vi "_PC_RTcheck rt_work_state.vi"(8 "error in (no error)":errorcluster, 11 "Stop":refnum<vi>) -> (0 "error out":errorcluster)   [LabVIEW 2018]
uses:
  RT/PublicSubVI/Ctl/_ctl_RT_Working_State.ctl
  <vilib>/Platform/TimedLoop/XDataNode/timing_clust.ctl
  <vilib>/Platform/TimedLoop/XDataNode/nitl_modes.ctl
  <vilib>/Platform/TimedLoop/XDataNode/wakeup.ctl
  <vilib>/Platform/TimedLoop/XDataNode/XDataNode.xnode
  <resource>/objmgr/ni.var.rc
  <vilib>/Platform/TimedLoop/XDataNode/XDNodeRunTimeDep.lvlib
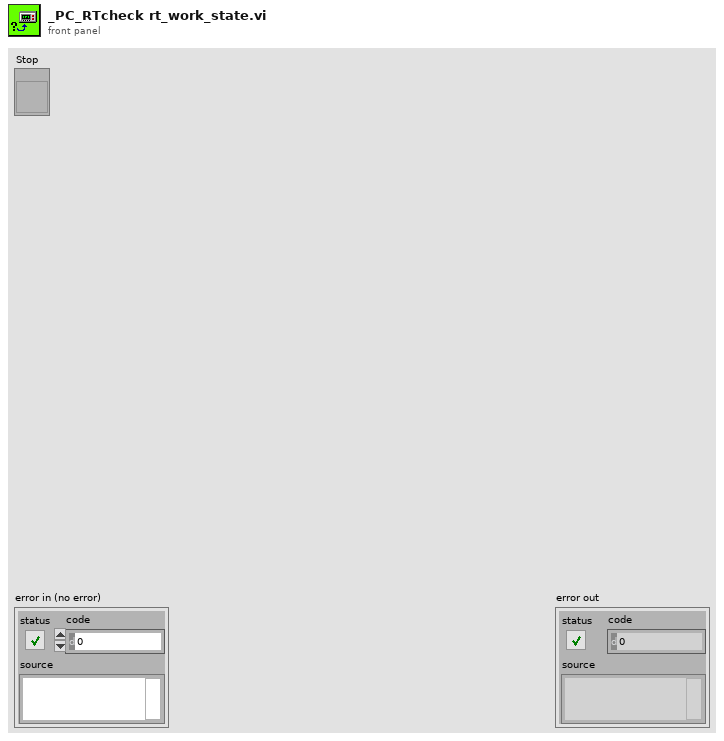
[diagram p1: front panel]
types:
  T1 = typedef "_ctl_RT_Working_State.ctl" = enum16{"Initialize", "Running", "Reboot_Work", "Reboot_Safe"}
  T2 = typedef "XDNodeRunTimeDep.lvlib/timing_clust.ctl" = cluster{"Expected End [f-1]":u64, "Actual End [f-1]":u64, "Finished Late? [f-1]":bool, "Expected End [i-1]":u64, "Actual End [i-1]":u64, "Finished Late? [i-1]":bool, "Expected Start [i]":u64, "Actual Start [i]":u64, "Expected Start [f]":u64, "Actual Start [f]":u64, "Source Name":string, "Structure Name":string, "Period":i64, "Deadline":i64, "Offset":i64, "Start":i64, "Priority":i32, "Timeout":i32, "Mode":T3, "Wakeup Reason":T4, "Error":errorcluster, "Source Type":string, "Secondary Source Type":string, "Global End Time":u64, "Global Start Time":u64, "Frame Duration":u64, "Iteration Duration":u64, "Assigned CPU":i32, "I/O Scan Engine Mode":u32}
  T3 = typedef "XDNodeRunTimeDep.lvlib/nitl_modes.ctl" = enum32{"No Change", "Process missed periods, maintain original phase", "Discard missed periods, maintain original phase", "Process missed periods, ignore original phase", "Discard missed periods, ignore original phase"}
  T4 = typedef "XDNodeRunTimeDep.lvlib/wakeup.ctl" = enum32{"Normal", "Aborted", "Asynchronous wakeup", "Timing source error", "Timed loop error", "Timeout"}
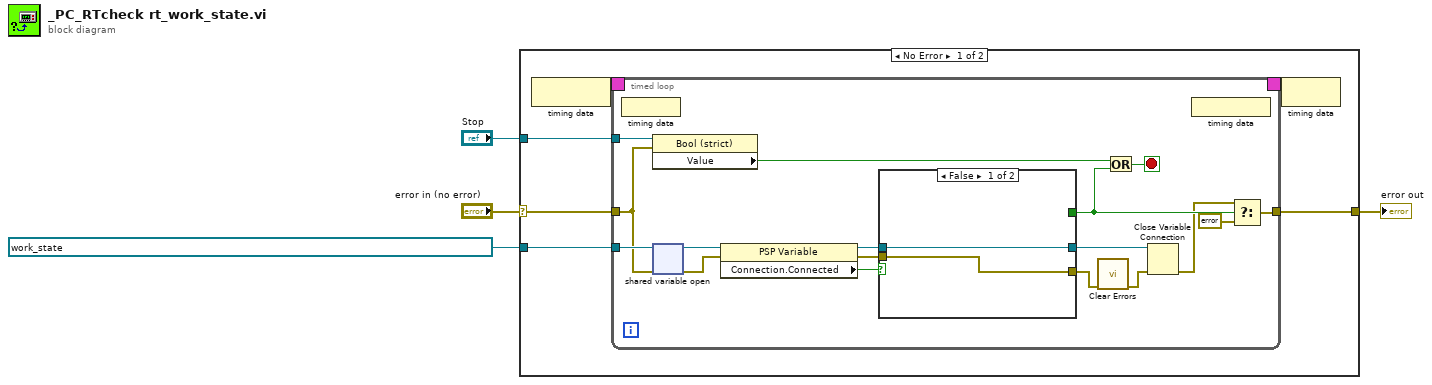
[diagram p0: block diagram]
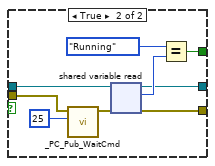
[diagram p2: hidden frame]
diagram:
  w3 = refnum<k21> "ni.var.psp://NI-sbRIO/_RT_CtrlLoop_Reboot_Monitor_Variable/RT_Working_State" items=["Initialize", "Running", "Reboot_Work", "Reboot_Safe"] ("shared variable refnum in")
  n1 = case shown="No Error" "error in (no error)" {
    selector: "error in (no error)" -> [w6 w43]
    tunnel: "Stop" -> [w8 _]
    tunnel: w3 -> [w7 _]
    tunnel: [w5 w43] -> w2
    frame No Error {
      n2 = node-c288() -> (w10:T2)
      n3 = timed-loop {
        tunnel: w8 -> [w27]
        timing: w10 -> [_]
        timing-out: [_] -> w9
        tunnel: w7 -> [w24]
        tunnel: [w12] -> w5
        tunnel: w6 -> [w11]
        stop <- w19 stop-if-true
        n4 = node-c288() -> ()  [unwired: 1 in]
        n5 = property class="Bool (strict)"(reference=w27, error in=w11) -> ("Value"=w20:bool)  [unwired: 2 out]
        n6 = shared-variable-open(w24, w11) -> (w26:refnum<k21>, w25:errorcluster)
        n7 = property class="PSP Variable"(reference=w26, error in=w25) -> (reference out=w23:refnum<k21>, error out=w21:errorcluster, "Connection.Connected"=w22:bool)
        n8 = case shown="False" w22 {
          tunnel: w23 -> [w29 w38]
          tunnel: w21 -> [w28 w37]
          tunnel: [_ w36] -> w15
          tunnel: [w28 w31] -> w16
          tunnel: [w29 w30] -> w17
          frame False {
          }
          frame True {
            n9 = call "_PC_Pub_WaitCmd.vi"("milliseconds to wait"=u32 25, "error in (no error)"=w37) -> ("error out"=w32:errorcluster)  [unwired: 9 in]
            n10 = shared-variable-read(w38, w32) -> (w30:refnum<k21>, w31:errorcluster, w35:T1)
            n11 = Equal?(x=_ctl_RT_Working_State."Running" ("y"), y=w35) -> (x = y?=w36:bool)
          }
        }
        n12 = call <vilib>:"Clear Errors.vi"("error in (no error)"=w16) -> ("error out"=w18:errorcluster)  [unwired: 5 in, 1 out]
        n13 = Or(x=w20, y=w15) -> (x .or. y?=w19:bool)
        n14 = Close Variable Connection(8:w18, 11:w17) -> (0:w14:errorcluster)
        n15 = node-c288() -> ()  [unwired: 1 out]
        n16 = Select(t=w14, s=w15, f=errorcluster {"status"=TRUE, "code"=7001, "source"="RT system response error"}) -> (s? t:f=w12:errorcluster)
      }
      n17 = node-c288(w9) -> ()
    }
    frame Error {
    }
  }
  "error out" <- w2
